vi "Stop Nested.vi"(10 "Error In":i32, 11 "Controller in":refnum<class "Controller.lvclass">) -> ()   [LabVIEW 2014]
uses:
  <userlib>/_Session Fwk/Session - Root.lvclass
  reusable/Session APIs/Session Log/System Log.lvclass
  Controller.lvclass
  Controls/Notifier Enum.ctl
panel:
  out "error out":errorcluster
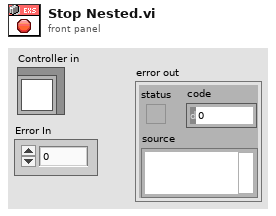
[diagram p1: front panel]
types:
  T1 = typedef "Controller.lvlib/Controller.lvclass/Notifier Enum.ctl" = enum16{"Initialize", "Get", "Set", "Close"}
  T2 = typedef "Session - Root.lvclass/Session Handle.ctl" = refnum<data-value>
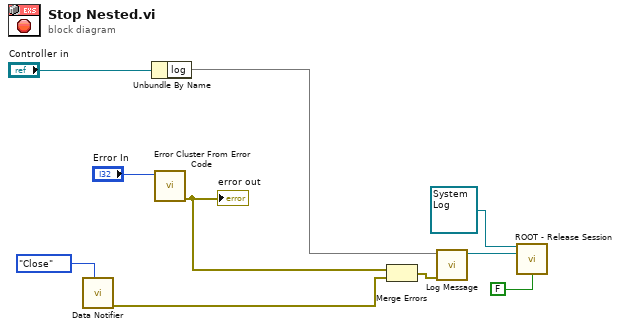
[diagram p0: block diagram]
diagram:
  n1 = call "Data Notifier.vi"("State"=Notifier_Enum."Close") -> ("error out"=w10:errorcluster)  [unwired: 9 in, 1 out]
  n2 = Unbundle By Name("Controller in") -> ("log"=w5)
  n3 = call <vilib>:"Error Cluster From Error Code.vi"("error code (0)"="Error In") -> ("error out"=w1:errorcluster)  [unwired: 8 in]
  "error out" <- w1
  n4 = Merge Errors(w1, w10) -> (w2:errorcluster)
  n5 = call "Log Message.vi"("error in"=w2, "session in"=w5) -> ("session out"=w6:T2)  [unwired: 8 in, 1 out]
  n6 = call <userlib>:"ROOT - Release Session.vi"("OBJ - Session in"=refnum<class "System Log.lvclass"> refnum ("Sys Log"), "Session Handle in"=w6, "force destroy? (F)"=FALSE) -> ()  [unwired: 11 in, 2 out]
